vi "Transverse_Set.vi"   [LabVIEW 2019]
uses:
  Globals/Climb_Globals.vi
  Climb_Transverse_Control_States.ctl
types:
  T1 = typedef "Climb_Transverse_Control_States.ctl" = enum16{"No-Op", "Manual", "Auto-Balancing"}
  T2 = typedef "Climb_Transverse_Cluster.ctl" = cluster{"Extend?":bool, "Transverse_Throttle":dbl, "Control_States":T1}
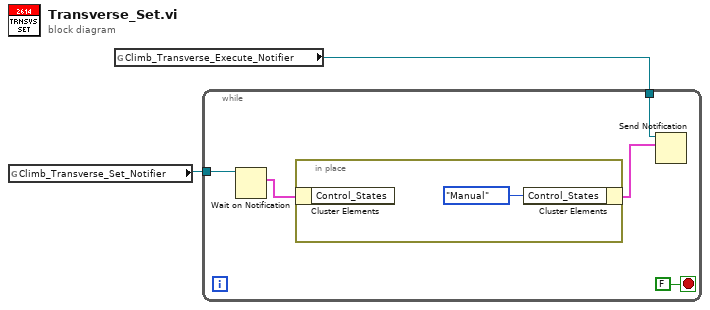
[diagram p0: block diagram]
diagram:
  n1 = global read "Climb_Globals.vi" "Climb_Transverse_Set_Notifier"() -> (w2:refnum<notifier>)
  n2 = global read "Climb_Globals.vi" "Climb_Transverse_Execute_Notifier"() -> (w1:refnum<notifier>)
  n3 = while {
    tunnel: w2 -> [w6]
    tunnel: w1 -> [w3]
    stop <- FALSE stop-if-true
    n4 = Wait on Notification(notifier=w6) -> (notification=w5:T2)  [unwired: 3 in, 3 out]
    n5 = in-place {
      n6 = in-place-cluster #1(w5) -> ()  [unwired: 1 out]
      n7 = in-place-cluster #1("Control_States"=Climb_Transverse_Control_States."Manual") -> (w4:T2)
    }
    n8 = Send Notification(notification=w4, notifier=w3) -> ()  [unwired: 1 in, 2 out]
  }
